vi "get channels test.vi"() -> ()   [LabVIEW 2013, in "OPC UA Server tests.lvlib"]
uses:
  OPC UA Server tests.lvlib
  module/configuration/OPC UA Server configuration.lvclass
panel:
  out "error out":errorcluster
  out "channels match":bool
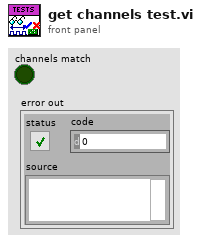
[diagram p1: front panel]
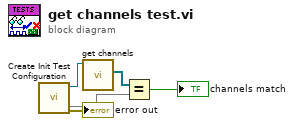
[diagram p0: block diagram]
diagram:
  n1 = call "Create Init Test Configuration.vi"() -> ("error out"=→"error out":errorcluster, "module"=w3:refnum<class "OPC UA Server configuration.lvclass">, 4:w1)  [unwired: 9 in]
  n2 = call-dynamic "get channels.vi"("OPC UA configuration in"=w3) -> ("channels"=w5:refnum<class "TBM channel.lvclass">[])  [unwired: 9 in, 1 out]
  n3 = Equal?(x=w5, y=w1) -> (x = y?=→"channels match":bool)
